vi "Einheit ersetzen.vi"(8 "Fehler (Eingang, kein Fehler)":errorcluster, 10 "Spaltentiitel":string, 11 "Einheit":string="[ppm]") -> (0 "Fehler (Ausgang)":errorcluster, 1 "offset past replacement":i32, 2 "number of replacements":i32, 3 "result string":string, 5 "Offset nach Übereinstimmung":i32)   [LabVIEW 2020, in "Linearisierung v2.lvlib"]
uses:
  Linearisierung v2.lvlib
  <vilib>/regexp/Match Regular Expression.xnode
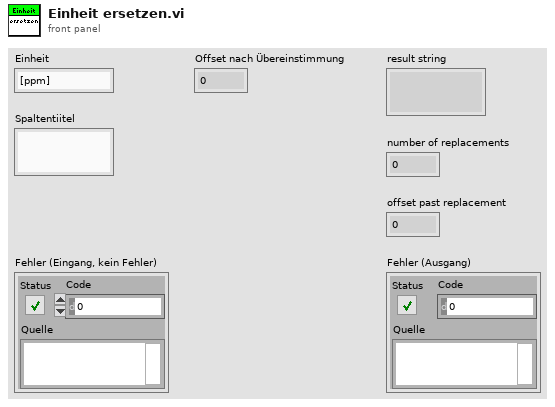
[diagram p1: front panel]
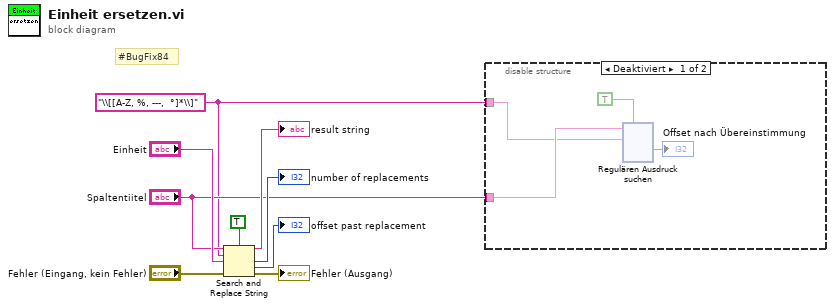
[diagram p0: block diagram]
diagram:
  w2 = "\\[[A-Z, %, ---,  °]*\\]" ("Such-String")
  # "#BugFix84"
  n1 = Search and Replace String(case sensitive?=TRUE ("Schreibweise ignorieren (F)"), input string="Spaltentiitel", search string=w2, replace string="Einheit", error in="Fehler (Eingang, kein Fehler)") -> (result string=→"result string":string, number of replacements=→"number of replacements":i32, offset past replacement=→"offset past replacement":i32, error out=→"Fehler (Ausgang)":errorcluster)  [unwired: 3 in]
  n2 = disable-structure shown="Deaktiviert" {
    disable-tunnel: "Spaltentiitel" -> [w13 _]
    disable-tunnel: w2 -> [w12 _]
    frame Disabled {
      n3 = xnode "Regulären Ausdruck suchen"("Eingangs-String"=w13, "Regulärer Ausdruck"=w12, "Schreibweise ignorieren (F)"=TRUE) -> ("Offset nach Übereinstimmung"=→"Offset nach Übereinstimmung":i32)  [unwired: 3 in, 4 out]
    }
    frame Enabled {
    }
  }
